vi "parse address.vi"(8 "error in (no error)":errorcluster, 10 "channel index":dbl) -> (0 "error out":errorcluster)   [LabVIEW 2020, in "TDK-Lambda Z.lvclass"]
uses:
  TDK-Lambda Z.lvclass
  TDK-Lambda Z.lvlib
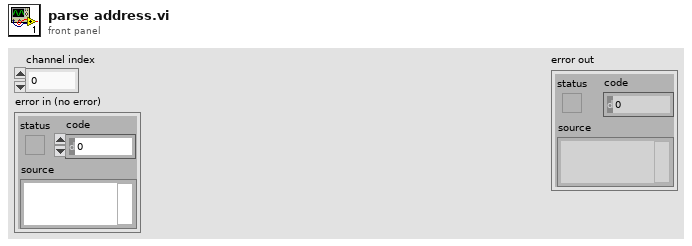
[diagram p1: front panel]
types:
  T1 = cluster{"setting.address.ch1":dbl, "setting.address.ch2":dbl, "setting.address.ch3":dbl, "setting.address.ch4":dbl, "visa resource name":string}
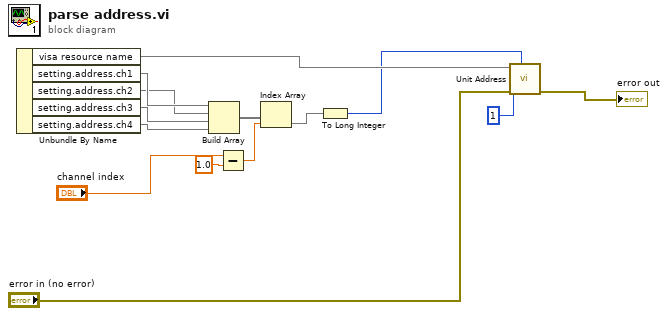
[diagram p0: block diagram]
diagram:
  n1 = Unbundle By Name() -> (w12:T1, "visa resource name"=w4, "setting.address.ch1"=w11, "setting.address.ch2"=w10, "setting.address.ch3"=w9, "setting.address.ch4"=w8)
  n2 = Build Array(w11, w10, w9, w8) -> (w15:void[])
  n3 = Subtract(x="channel index", y=1.0 ("x")) -> (x-y=w13:dbl)
  n4 = Index Array(array=w15, index=w13) -> (element=w6)
  n5 = To Long Integer(number=w6) -> (32bit integer=w3:i32)
  n6 = call "Unit Address.vi"("Address (6)"=w3, "error in (no error)"="error in (no error)", "Language Selector (-1)"=i16 1 ("Address (6)"), "VISA resource name"=w4) -> ("error out"=→"error out":errorcluster)  [unwired: 6 in, 1 out]
